vi "Zebra zt230 barcode printer.vi"(6 "error in":errorcluster) -> (0 "error out":errorcluster, 1 "Final Serial No":string, 3 "prn file":string="<xpml><page quantity='0' pitch='20.1 mm'></xpml>SIZE 39.10 mm, 20.1 mm\nGAP 3 mm, 0 mm\nDIRECTION 0,0\nREFERENCE 0,0\nOFFSET 0 mm\nSET PEEL OFF\nSET CUTTER OFF\nSET PARTIAL_CUTTER OFF\n<xpml></page></xpml><xpml><page quantity='1' pitch='20.1 mm'></xpml>SET TEAR ON\nCLS\nCODEPAGE 1252\nTEXT 445,152,\"0\",180,56,30,\"4\"\nTEXT 447,200,\"0\",180,6,6,\"JKT.COL.STRG.ASSY (48810 640B0)\"\nTEXT 328,150,\"0\",180,6,6,\"45250-0K100\"\nQRCODE 164,159,L,7,A,180,M2,S7,\"4-45250-0K100-161006-A\"\nTEXT 448,37,\"0\",180,6,6,\"16.11.19-A  SFAL\"\nPRINT 1,1\n<xpml></page></xpml><xpml><end/></xpml>")   [LabVIEW 2015]
panel:
  out "length":i32
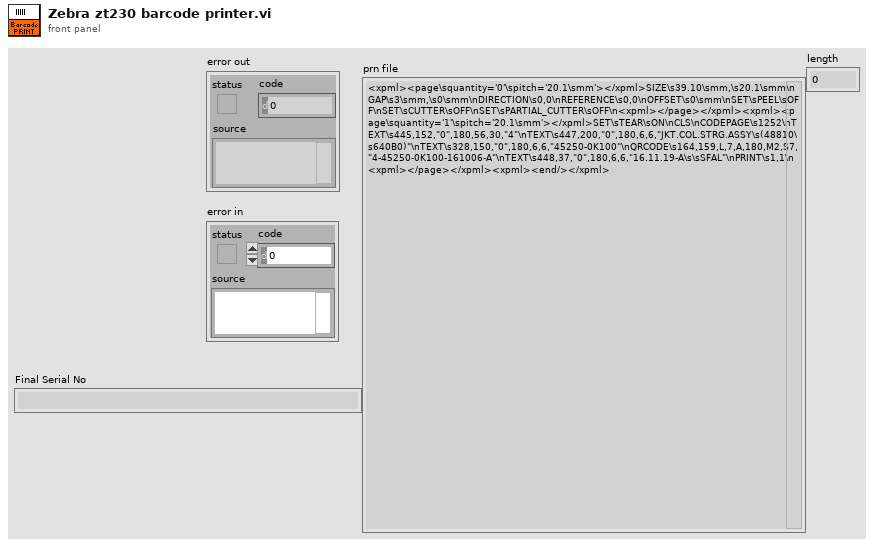
[diagram p1: front panel]
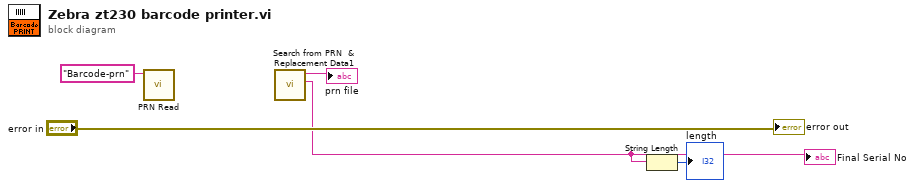
[diagram p0: block diagram]
diagram:
  n1 = call "PRN Read.vi"("prn"="Barcode-prn") -> ()  [unwired: 9 in, 2 out]
  n2 = call "Search from PRN  & Replacement Data1.vi"() -> ("send on  barcode printer"=→"prn file":string, "Barcode Serial No"=w2:string)  [unwired: 9 in]
  "Final Serial No" <- w2
  n3 = String Length(string=w2) -> (length=→"length":i32)
  "error out" <- "error in"
